vi "Set Frequency Mode.vi"(8 "error in (no error)":errorcluster, 9 "Mode (0: CW)":T1, 10 "Channel (0: Channel 1)":T2 items=["Channel 1", "Channel 2"], 11 "VISA resource name":refnum<visa-resource-name>) -> (0 "error out":errorcluster, 3 "VISA resource name out":refnum<visa-resource-name>)   [LabVIEW 2009, in "Tektronix AFG 3000 Series.lvlib"]
doc: "Sets the frequency mode (sweep vs. continuous) of a Tektronix AFG 3000 series function generator."
uses:
  Tektronix AFG 3000 Series.lvlib
  controls.llb/Channel.ctl
  controls.llb/Frequency Mode.ctl
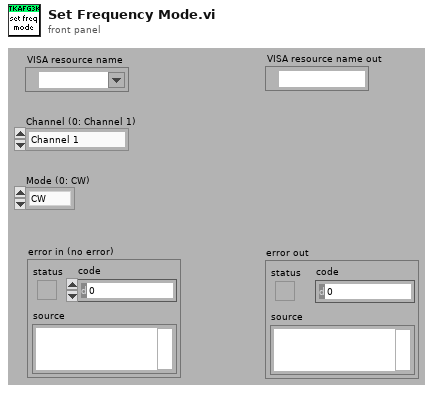
[diagram p1: front panel]
types:
  T1 = typedef "Frequency Mode.ctl" = enum16{"CW", "Sweep"}
  T2 = typedef "Channel.ctl" = u16
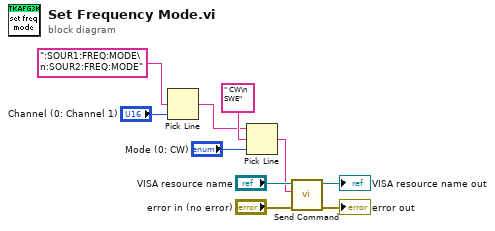
[diagram p0: block diagram]
diagram:
  n1 = Pick Line(multi-line string=":SOUR1:FREQ:MODE\n:SOUR2:FREQ:MODE", line index="Channel (0: Channel 1)") -> (output string=w3:string)  [unwired: 1 out]
  n2 = Pick Line(string ("")=w3, multi-line string=" CW\n SWE", line index="Mode (0: CW)") -> (output string=w1:string)
  n3 = call "Send Command.vi"("error in (no error)"="error in (no error)", "write buffer"=w1, "VISA resource name"="VISA resource name") -> ("error out"=→"error out":errorcluster, "VISA resource name out"=→"VISA resource name out":refnum<visa-resource-name>)  [unwired: 7 out]
